vi "Diff_Drive_System_Get_Distance.vi"() -> (1 "Right Distance FT":dbl, 3 "Left Distance FT":dbl)   [LabVIEW 2019]
uses:
  Diff_Drive_System_Globals.vi
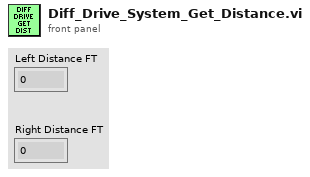
[diagram p1: front panel]
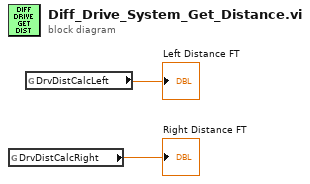
[diagram p0: block diagram]
diagram:
  n1 = global read "Diff_Drive_System_Globals.vi" "DrvDistCalcRight"() -> (→"Right Distance FT":dbl)
  n2 = global read "Diff_Drive_System_Globals.vi" "DrvDistCalcLeft"() -> (→"Left Distance FT":dbl)
